vi "Extract +ve and -ve Current Readings.vi"(10 "Input Array":dbl[](array[numeric])=[6.0, 3.9, -5.8, 0.0, -2.6, -1.0, 2.2, -4.3] format="%0.2f") -> (0 "Negative Current":dbl[](array[numeric]) format="%0.2f", 3 "Positive Current":dbl[](array[numeric]) format="%0.2f")   [LabVIEW 2010]
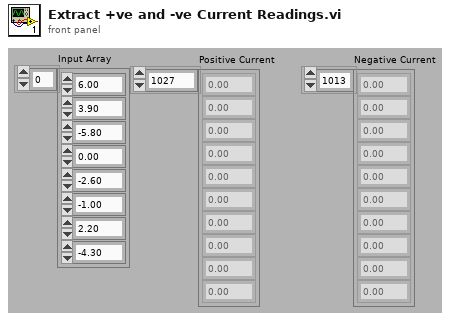
[diagram p1: front panel]
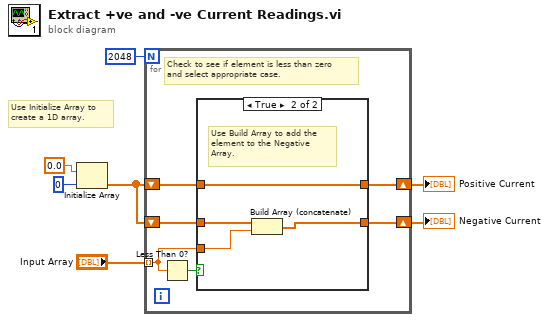
[diagram p0: block diagram]
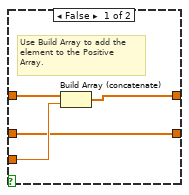
[diagram p2: hidden frame]
diagram:
  # "Use Initialize Array to\ncreate a 1D array."
  n1 = Initialize Array(0.0, 0) -> (w3:dbl[])
  n2 = for {
    N: 2048 -> [_]
    shift-right: [w11] -> w6
    shift-left: w3 -> [w10]
    shift-right: [w8] -> w7
    shift-left: w3 -> [w9]
    tunnel: "Input Array" -> [w12] mode=indexing
    # "Check to see if element is less than zero\nand select appropriate case."
    n3 = Less Than 0?(x=w12) -> (x < 0?=w13:bool)
    n4 = case shown="True" w13 {
      tunnel: w12 -> [w15 w20]
      tunnel: [w16 w21] -> w11
      tunnel: w10 -> [w17 w21]
      tunnel: w9 -> [w14 w19]
      tunnel: [w14 w18] -> w8
      frame False {
        # "Use Build Array to add the\nelement to the Positive\nArray."
        n5 = Build Array (concatenate)(w17, w15) -> (w16:dbl[])
      }
      frame True {
        # "Use Build Array to add the\nelement to the Negative\nArray."
        n6 = Build Array (concatenate)(w19, w20) -> (w18:dbl[])
      }
    }
  }
  "Positive Current" <- w6
  "Negative Current" <- w7
